vi "Secondary System - Gamepad.vi"() -> (2 "Arm Height Setting":dbl)   [LabVIEW 2011]
panel:
  in  "Arm Constants":T1={"Top Center Peg"=166.0, "Top Outer Pegs"=155.0, "Middle Center Peg"=118.0, "Middle Outer Pegs"=109.0, "Lower Center Peg"=76.0, "Lower Outside Pegs"=73.0, "Feed"=20.0, "Floor"=13.0}
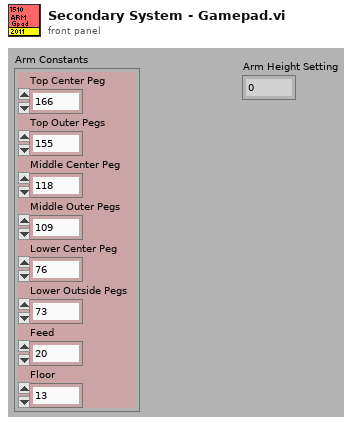
[diagram p1: front panel]
types:
  T1 = cluster{"Top Center Peg":dbl, "Top Outer Pegs":dbl, "Middle Center Peg":dbl, "Middle Outer Pegs":dbl, "Lower Center Peg":dbl, "Lower Outside Pegs":dbl, "Feed":dbl, "Floor":dbl}
  T2 = typedef "Arm Joystick.ctl" = cluster{"Buttons":T3, "Axes":cluster{"axis 1 (x)":dbl, "axis 2 (y)":dbl, "axis 3 (throttle)":dbl, "axis 4":dbl, "axis 5":dbl, "axis 6":dbl}}
  T3 = typedef "WPI_JoystickButtonState.ctl" = cluster{"Button 1":bool, "Button 2":bool, "Button 3":bool, "Button 4":bool, "Button 5":bool, "Button 6":bool, "Button 7":bool, "Button 8":bool, "Button 9":bool, "Button 10":bool, "Button 11":bool, "Button 12":bool}
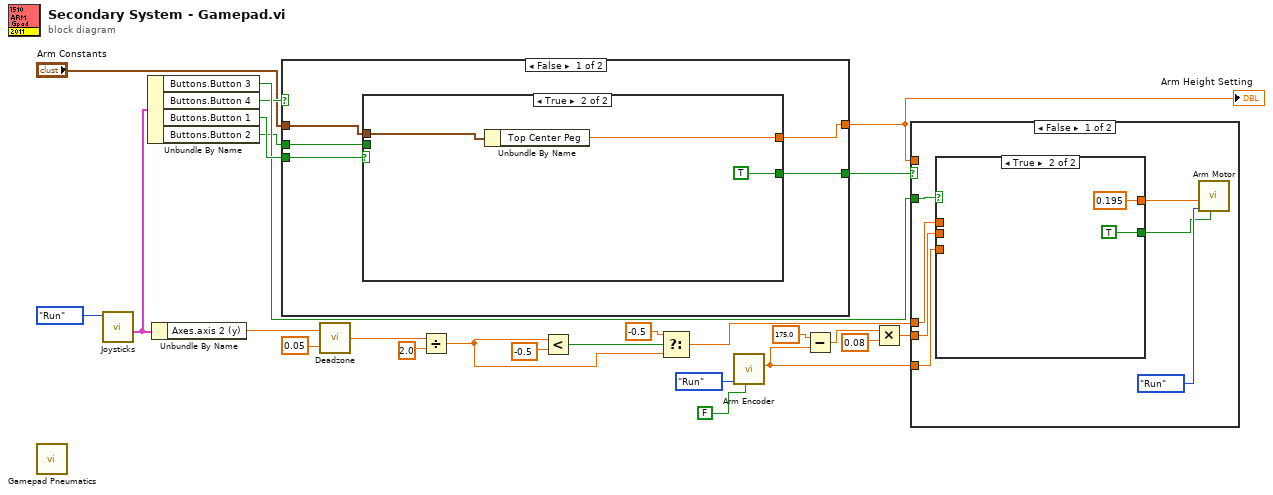
[diagram p0: block diagram]
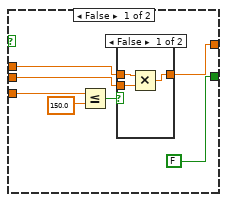
[diagram p2: hidden frame]
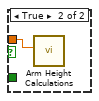
[diagram p4: hidden frame]
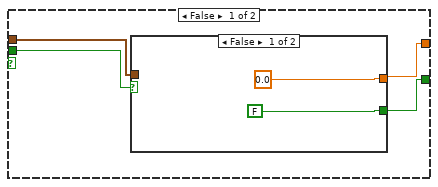
[diagram p5: hidden frame]
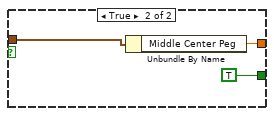
[diagram p6: hidden frame]
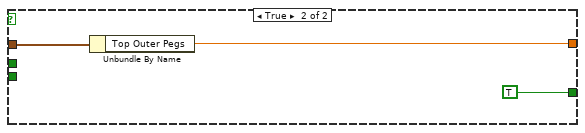
[diagram p7: hidden frame]
diagram:
  n1 = call "Gamepad Pneumatics.vi"() -> ()  [unwired: 1 out]
  n2 = call "Joysticks.vi"("Mode"=enum16{"Init", "Run", "End"}."Run") -> ("Arm Joystick"=w23:T2)  [unwired: 8 out]
  n3 = Unbundle By Name(w23) -> ("Buttons.Button 3"=w17:bool, "Buttons.Button 4"=w14:bool, "Buttons.Button 1"=w25:bool, "Buttons.Button 2"=w15:bool)
  n4 = Unbundle By Name(w23) -> ("Axes.axis 2 (y)"=w2:dbl)
  n5 = case shown="False" w14 {
    tunnel: [w29 TRUE] -> w16
    tunnel: [w30 w43] -> w13
    tunnel: w25 -> [w28 _]
    tunnel: w15 -> [w27 _]
    tunnel: "Arm Constants" -> [w26 w44]
    frame False {
      n6 = case shown="True" w28 {
        tunnel: [w33 w41] -> w30
        tunnel: [w34 TRUE] -> w29
        tunnel: w27 -> [w32 _]
        tunnel: w26 -> [w31 w40]
        frame False {
          n7 = case shown="False" w32 {
            tunnel: [FALSE TRUE] -> w34
            tunnel: [0.0 ("Middle Outer Pegs") w37] -> w33
            tunnel: w31 -> [_ w38]
            frame False {
            }
            frame True {
              n8 = Unbundle By Name(w38) -> ("Middle Center Peg"=w37:dbl)
            }
          }
        }
        frame True {
          n9 = Unbundle By Name(w40) -> ("Top Center Peg"=w41:dbl)
        }
      }
    }
    frame True {
      n10 = Unbundle By Name(w44) -> ("Top Outer Pegs"=w43:dbl)
    }
  }
  "Arm Height Setting" <- w13
  n11 = call "Deadzone.vi"("Deadzone"=0.05, "Input"=w2) -> ("Output"=w1:dbl)
  n12 = Divide(x=w1, y=2.0) -> (x/y=w7:dbl)
  n13 = Less?(x=w7, y=-0.5) -> (x < y?=w9:bool)
  n14 = Select(t=-0.5, s=w9, f=w7) -> (s? t:f=w6:dbl)
  n15 = call "Arm Encoder.vi"("Reset Encoder?"=FALSE, "Mode"=enum16{"Init", "Run", "End"}."Run") -> ("Get Arm Encoder"=w12:dbl)  [unwired: 1 in, 8 out]
  n16 = Subtract(x=175.0, y=w12) -> (x-y=w18:dbl)
  n17 = Multiply(x=w18, y=0.08) -> (x*y=w20:dbl)
  n18 = case shown="False" w16 {
    tunnel: w17 -> [w49 _]
    tunnel: w12 -> [w52 _]
    tunnel: w6 -> [w51 _]
    tunnel: w20 -> [w50 _]
    tunnel: w13 -> [_ w66]
    frame False {
      n19 = case shown="True" w49 {
        tunnel: w52 -> [w59 _]
        tunnel: w51 -> [w57 _]
        tunnel: w50 -> [w56 _]
        tunnel: [w55 0.195] -> w47
        tunnel: [FALSE TRUE] -> w46
        frame False {
          n20 = Less Or Equal?(x=w59, y=150.0) -> (x <= y?=w58:bool)
          n21 = case shown="False" w58 {
            tunnel: w57 -> [w62 w63]
            tunnel: [w60 w63] -> w55
            tunnel: w56 -> [w61 _]
            frame False {
              n22 = Multiply(x=w62, y=w61) -> (x*y=w60:dbl)
            }
            frame True {
            }
          }
        }
        frame True {
        }
      }
      n23 = call "Arm Motor.vi"("Stall Arm?"=w46, "Mode"=enum16{"Init", "Run", "End"}."Run", "Arm motor speed"=w47) -> ()  [unwired: 1 in, 8 out]
    }
    frame True {
      n24 = call "Arm Height Calculations.vi"("Height Input"=w66) -> ()  [unwired: 11 out]
    }
  }
